vi "Sort Song Dysplay.vi"(7 "Options":T1, 8 "Error In":errorcluster, 10 "Reverse?":bool, 11 "Songs":T2[](array[typedef]) {"Duration (s)" format="%<%M:%S>T"}) -> (0 "Error Out":errorcluster, 3 "Sorted Songs":T2[](array[typedef]) {"Duration (s)" format="%<%M:%S>T"})   [LabVIEW 2015]
uses:
  app/controls/Queue Song Display.ctl
  MusicElement/Song/Song Duration.ctl
  app/controls/Dequeue Control.ctl
  Song Display Sort Option.ctl
  MusicElement/Song/Song.lvclass
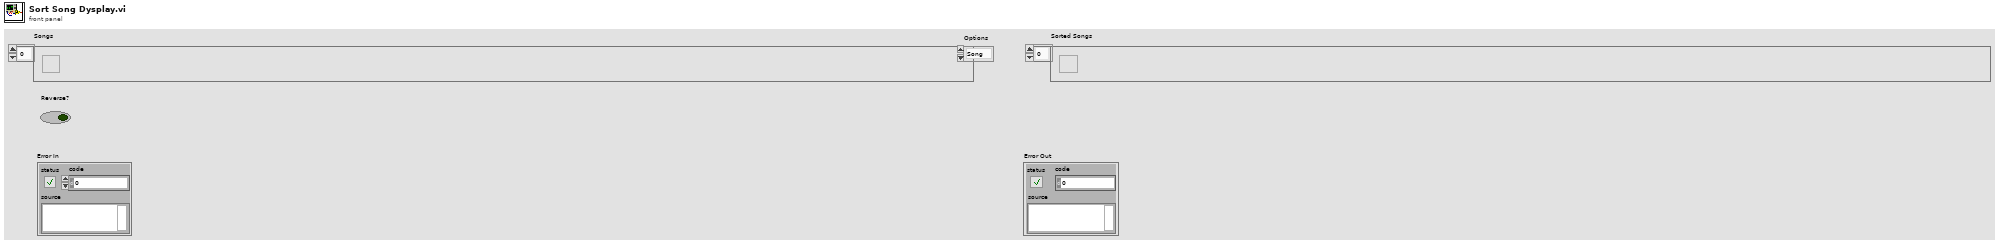
[diagram p1: front panel]
types:
  T1 = typedef "Song Display Sort Option.ctl" = enum16{"Song", "Artist", "Album", "Time"}
  T2 = typedef "Queue Song Display.ctl" = cluster{"Song Name":string, "Artist":string, "Album":string, "Duration (s)":T3, "UID":string, "Dequeue":T4}
  T3 = typedef "Song.lvclass/Song Duration.ctl" = timestamp
  T4 = typedef "Dequeue Control.ctl" = bool
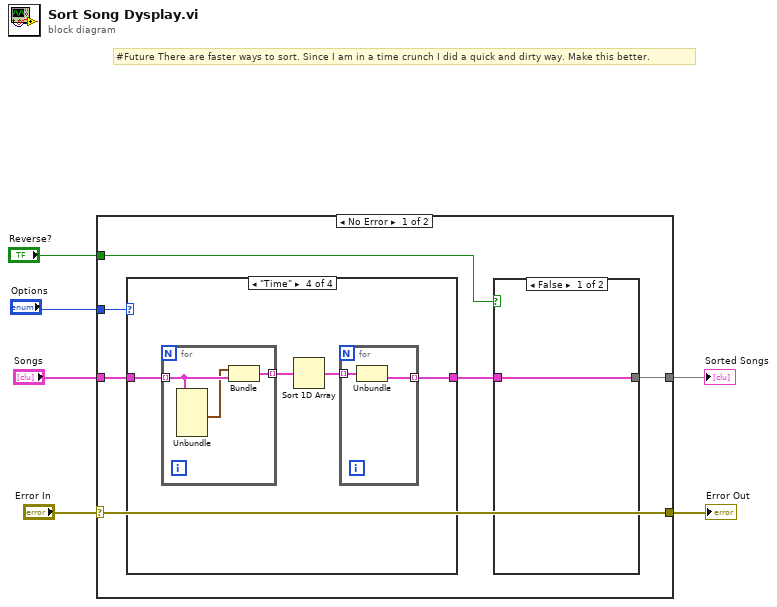
[diagram p0: block diagram]
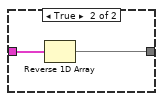
[diagram p2: hidden frame]
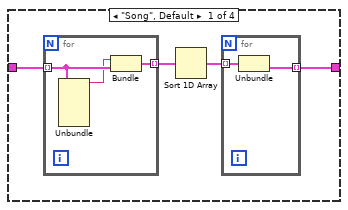
[diagram p3: hidden frame]
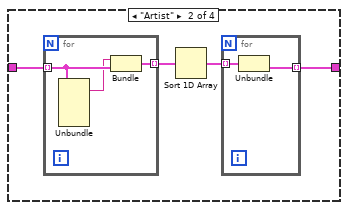
[diagram p4: hidden frame]
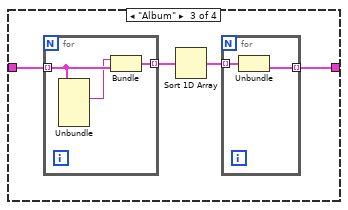
[diagram p5: hidden frame]
diagram:
  # "#Future There are faster ways to sort. Since I am in a time crunch I did a quick and dirty way. Make this better."
  n1 = case shown="No Error" "Error In" {
    selector: "Error In" -> [w8 w53]
    tunnel: [w8 w53] -> w5
    tunnel: "Songs" -> [w11 w52]
    tunnel: "Options" -> [w12 _]
    tunnel: "Reverse?" -> [w10 _]
    tunnel: [w7 w52] -> w2
    frame No Error {
      n2 = case shown="\"Time\"" w12 {
        tunnel: w11 -> [w19 w28 w37 w46]
        tunnel: [w16 w25 w34 w43] -> w9
        frame "Song", Default {
          n3 = for {
            tunnel: w19 -> [w24] mode=indexing
            tunnel: [w23] -> w18 mode=indexing
            n4 = Unbundle(w24) -> ("Song Name"=w22:string)  [unwired: 5 out]
            n5 = Bundle("Song Name"=w22, "Sorted Song"=w24) -> (w23:cluster{"Song Name":string, "Sorted Song":T2})  [unwired: 1 in]
          }
          n6 = Sort 1D Array(array=w18) -> (sorted array=w17:cluster{"Song Name":string, "Sorted Song":T2}[])
          n7 = for {
            tunnel: w17 -> [w21] mode=indexing
            tunnel: [w20] -> w16 mode=indexing
            n8 = Unbundle(w21) -> ("Sorted Song"=w20:T2)  [unwired: 1 out]
          }
        }
        frame "Artist" {
          n9 = for {
            tunnel: w28 -> [w33] mode=indexing
            tunnel: [w32] -> w27 mode=indexing
            n10 = Unbundle(w33) -> ("Artist"=w31:string)  [unwired: 5 out]
            n11 = Bundle("Artist"=w31, "Sorted Song"=w33) -> (w32:cluster{"Artist":string, "Sorted Song":T2})  [unwired: 1 in]
          }
          n12 = Sort 1D Array(array=w27) -> (sorted array=w26:cluster{"Artist":string, "Sorted Song":T2}[])
          n13 = for {
            tunnel: w26 -> [w30] mode=indexing
            tunnel: [w29] -> w25 mode=indexing
            n14 = Unbundle(w30) -> ("Sorted Song"=w29:T2)  [unwired: 1 out]
          }
        }
        frame "Album" {
          n15 = for {
            tunnel: w37 -> [w42] mode=indexing
            tunnel: [w41] -> w36 mode=indexing
            n16 = Unbundle(w42) -> ("Album"=w40:string)  [unwired: 5 out]
            n17 = Bundle("Album"=w40, "Sorted Song"=w42) -> (w41:cluster{"Album":string, "Sorted Song":T2})  [unwired: 1 in]
          }
          n18 = Sort 1D Array(array=w36) -> (sorted array=w35:cluster{"Album":string, "Sorted Song":T2}[])
          n19 = for {
            tunnel: w35 -> [w39] mode=indexing
            tunnel: [w38] -> w34 mode=indexing
            n20 = Unbundle(w39) -> ("Sorted Song"=w38:T2)  [unwired: 1 out]
          }
        }
        frame "Time" {
          n21 = for {
            tunnel: w46 -> [w51] mode=indexing
            tunnel: [w50] -> w45 mode=indexing
            n22 = Unbundle(w51) -> ("Duration (s)"=w49:T3)  [unwired: 5 out]
            n23 = Bundle("Duration (s)"=w49, "Sorted Song"=w51) -> (w50:cluster{"Duration (s)":T3, "Sorted Song":T2})  [unwired: 1 in]
          }
          n24 = Sort 1D Array(array=w45) -> (sorted array=w44:cluster{"Duration (s)":T3, "Sorted Song":T2}[])
          n25 = for {
            tunnel: w44 -> [w48] mode=indexing
            tunnel: [w47] -> w43 mode=indexing
            n26 = Unbundle(w48) -> ("Sorted Song"=w47:T2)  [unwired: 1 out]
          }
        }
      }
      n27 = case shown="False" w10 {
        tunnel: w9 -> [w13 w15]
        tunnel: [w13 w14] -> w7
        frame False {
        }
        frame True {
          n28 = Reverse 1D Array(array=w15) -> (reversed array=w14:T2[])
        }
      }
    }
    frame Error {
    }
  }
  "Error Out" <- w5
  "Sorted Songs" <- w2
